vi "Configure I2C.vi"(8 "error in (no error)":errorcluster, 9 "I2C Message Byte":u8[](array[numeric]) format="%.0x", 10 "I2C Address (0)":u8, 11 "VISA resource name":refnum<visa-resource-name>) -> (0 "error out":errorcluster, 3 "VISA resource name out":refnum<visa-resource-name>)   [LabVIEW 2021, in "Ocean Optics 2000 4000.lvlib"]
doc: "Configures the I2C (Inter-Integrated Circuit) on the spectrometer for interfacing to attached peripherals. The I2C bus runs at 400kHz."
uses:
  <instrlib>/Ocean Optics 2000 4000/Ocean Optics 2000 4000.lvlib
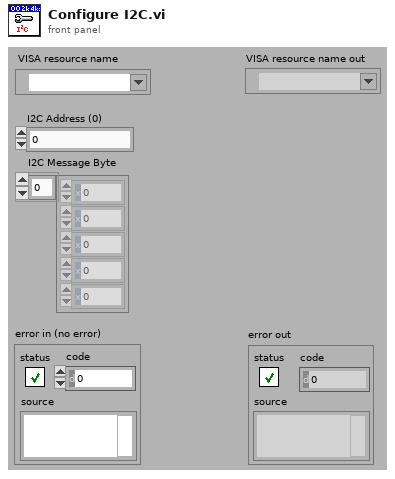
[diagram p1: front panel]
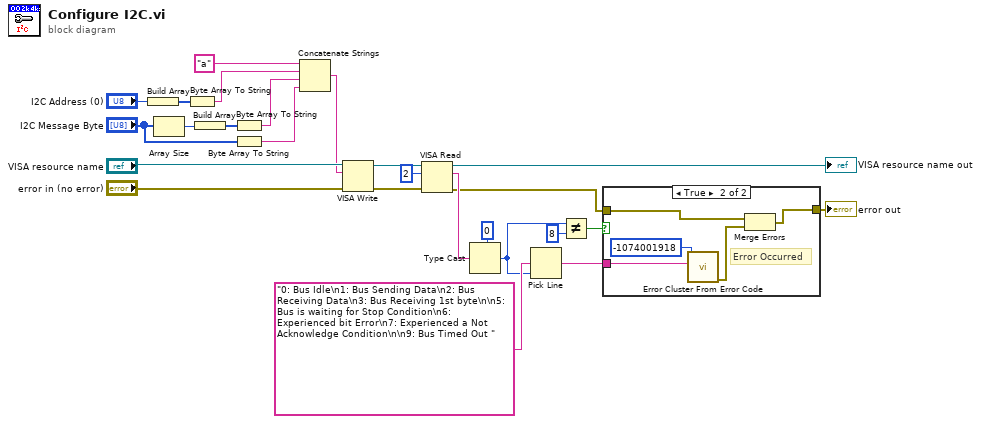
[diagram p0: block diagram]
diagram:
  n1 = Build Array("I2C Address (0)") -> (w21:u8[])
  n2 = Array Size(array="I2C Message Byte") -> (size(s)=w18:i32)
  n3 = Byte Array To String(unsigned byte array=w21) -> (string=w20:string)
  n4 = Build Array(w18) -> (w19:i32[])
  n5 = Byte Array To String(unsigned byte array=w19) -> (string=w17:string)
  n6 = Byte Array To String(unsigned byte array="I2C Message Byte") -> (string=w15:string)
  n7 = Concatenate Strings("a" ("string"), w20, w17, w15) -> (w14:string)
  n8 = VISA Write(VISA resource name="VISA resource name", write buffer=w14, error in (no error)="error in (no error)") -> (VISA resource name out=w12:refnum<visa-resource-name>, error out=w11:errorcluster)  [unwired: 1 out]
  n9 = VISA Read(VISA resource name=w12, byte count=u32 2, error in (no error)=w11) -> (VISA resource name out=→"VISA resource name out":refnum<visa-resource-name>, read buffer=w9:string, error out=w3:errorcluster)  [unwired: 1 out]
  n10 = Type Cast(type=u8 0, x=w9) -> (*(type *) &x=w1:u8)
  n11 = Pick Line(multi-line string="0: Bus Idle\n1: Bus Sending Data\n2: Bus Receiving Data\n3: Bus Receiving 1st byte\n\n5: Bus is waiting for Stop Condition\n6: Experienced bit Error\n7: Experienced a Not Acknowledge Condition\n\n9: Bus Timed Out ", line index=w1) -> (output string=w6:string)  [unwired: 1 out]
  n12 = Not Equal?(x=w1, y=u8 8) -> (x != y?=w5:bool)
  n13 = case shown="True" w5 {
    tunnel: w6 -> [_ w31]
    tunnel: w3 -> [w26 w28]
    tunnel: [w26 w27] -> w2
    frame False {
      # "No Error"
    }
    frame True {
      # "Error Occurred"
      n14 = call <vilib>:"Error Cluster From Error Code.vi"("error message (\"\")"=w31, "error code (0)"=-1074001918) -> ("error out"=w29:errorcluster)  [unwired: 2 in, 5 out]
      n15 = Merge Errors(w28, w29) -> (w27:errorcluster)
    }
  }
  "error out" <- w2
